vi "Setattribute_value.vi"(8 "error in (no error)":errorcluster, 10 "Set_Val":T1, 11 "OneOfTemplate in":refnum<class "niswitch_grpc_SetAttributeViInt32Request_attribute_value_enum.lvclass">) -> (0 "error out":errorcluster, 3 "OneOfTemplate out":refnum<class "niswitch_grpc_SetAttributeViInt32Request_attribute_value_enum.lvclass">)   [LabVIEW 2021, in "NI Switch_client.lvlib" / "niswitch_grpc_SetAttributeViInt32Request_attribute_value_enum.lvclass"]
uses:
  niswitch_grpc_SetAttributeViInt32Request_attribute_value_enum.lvclass
  niswitch_grpc_NiSwitchInt32AttributeValues.ctl
  niswitch_grpc_SetAttributeViInt32Request_attribute_value_enum.lvclass/niswitch_grpc_SetAttributeViInt32Request_attribute_value_enum.ctl
  NI Switch_client.lvlib
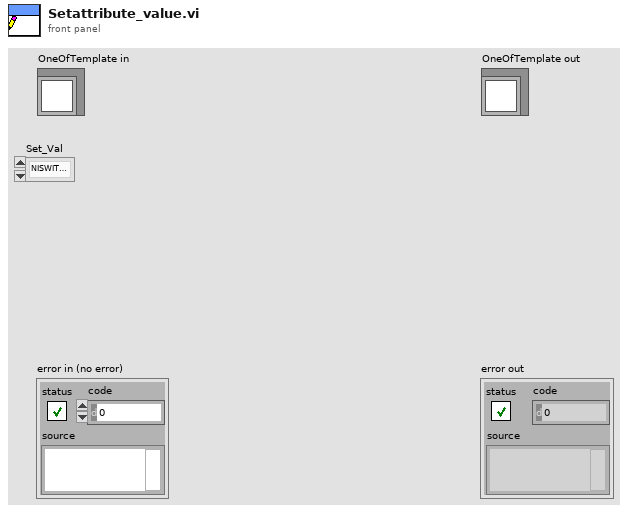
[diagram p1: front panel]
types:
  T1 = typedef "NI Switch_client.lvlib/niswitch_grpc_NiSwitchInt32AttributeValues.ctl" = enum32{"NISWITCH_INT32_UNSPECIFIED", "NISWITCH_INT32_HANDSHAKING_INITIATION_VAL_MEASUREMENT_DEVICE_INITIATED", "NISWITCH_INT32_HANDSHAKING_INITIATION_VAL_SWITCH_INITIATED", "NISWITCH_INT32_SCAN_ADVANCED_OUTPUT_VAL_NONE", "NISWITCH_INT32_SCAN_ADVANCED_OUTPUT_VAL_EXTERNAL", "NISWITCH_INT32_SCAN_ADVANCED_OUTPUT_VAL_TTL0", "NISWITCH_INT32_SCAN_ADVANCED_OUTPUT_VAL_TTL1", "NISWITCH_INT32_SCAN_ADVANCED_OUTPUT_VAL_TTL2", "NISWITCH_INT32_SCAN_ADVANCED_OUTPUT_VAL_TTL3", "NISWITCH_INT32_SCAN_ADVANCED_OUTPUT_VAL_TTL4", "NISWITCH_INT32_SCAN_ADVANCED_OUTPUT_VAL_TTL5", "NISWITCH_INT32_SCAN_ADVANCED_OUTPUT_VAL_TTL6", "NISWITCH_INT32_SCAN_ADVANCED_OUTPUT_VAL_TTL7", "NISWITCH_INT32_SCAN_ADVANCED_OUTPUT_VAL_PXI_STAR", "NISWITCH_INT32_SCAN_ADVANCED_OUTPUT_VAL_REARCONNECTOR", "NISWITCH_INT32_SCAN_ADVANCED_OUTPUT_VAL_FRONTCONNECTOR", "NISWITCH_INT32_SCAN_ADVANCED_OUTPUT_VAL_REARCONNECTOR_MODULE1", "NISWITCH_INT32_SCAN_ADVANCED_OUTPUT_VAL_REARCONNECTOR_MODULE2", "NISWITCH_INT32_SCAN_ADVANCED_OUTPUT_VAL_REARCONNECTOR_MODULE3", "NISWITCH_INT32_SCAN_ADVANCED_OUTPUT_VAL_REARCONNECTOR_MODULE4", "NISWITCH_INT32_SCAN_ADVANCED_OUTPUT_VAL_REARCONNECTOR_MODULE5", "NISWITCH_INT32_SCAN_ADVANCED_OUTPUT_VAL_REARCONNECTOR_MODULE6", "NISWITCH_INT32_SCAN_ADVANCED_OUTPUT_VAL_REARCONNECTOR_MODULE7", "NISWITCH_INT32_SCAN_ADVANCED_OUTPUT_VAL_REARCONNECTOR_MODULE8", "NISWITCH_INT32_SCAN_ADVANCED_OUTPUT_VAL_REARCONNECTOR_MODULE9", "NISWITCH_INT32_SCAN_ADVANCED_OUTPUT_VAL_REARCONNECTOR_MODULE10", "NISWITCH_INT32_SCAN_ADVANCED_OUTPUT_VAL_REARCONNECTOR_MODULE11", "NISWITCH_INT32_SCAN_ADVANCED_OUTPUT_VAL_REARCONNECTOR_MODULE12", "NISWITCH_INT32_SCAN_ADVANCED_OUTPUT_VAL_FRONTCONNECTOR_MODULE1", "NISWITCH_INT32_SCAN_ADVANCED_OUTPUT_VAL_FRONTCONNECTOR_MODULE2", "NISWITCH_INT32_SCAN_ADVANCED_OUTPUT_VAL_FRONTCONNECTOR_MODULE3", "NISWITCH_INT32_SCAN_ADVANCED_OUTPUT_VAL_FRONTCONNECTOR_MODULE4", "NISWITCH_INT32_SCAN_ADVANCED_OUTPUT_VAL_FRONTCONNECTOR_MODULE5", "NISWITCH_INT32_SCAN_ADVANCED_OUTPUT_VAL_FRONTCONNECTOR_MODULE6", "NISWITCH_INT32_SCAN_ADVANCED_OUTPUT_VAL_FRONTCONNECTOR_MODULE7", "NISWITCH_INT32_SCAN_ADVANCED_OUTPUT_VAL_FRONTCONNECTOR_MODULE8", "NISWITCH_INT32_SCAN_ADVANCED_OUTPUT_VAL_FRONTCONNECTOR_MODULE9", "NISWITCH_INT32_SCAN_ADVANCED_OUTPUT_VAL_FRONTCONNECTOR_MODULE10", "NISWITCH_INT32_SCAN_ADVANCED_OUTPUT_VAL_FRONTCONNECTOR_MODULE11", "NISWITCH_INT32_SCAN_ADVANCED_OUTPUT_VAL_FRONTCONNECTOR_MODULE12", "NISWITCH_INT32_SCAN_ADVANCED_POLARITY_VAL_RISING_EDGE", "NISWITCH_INT32_SCAN_ADVANCED_POLARITY_VAL_FALLING_EDGE", "NISWITCH_INT32_SCAN_MODE_VAL_NONE", "NISWITCH_INT32_SCAN_MODE_VAL_BREAK_BEFORE_MAKE", "NISWITCH_INT32_SCAN_MODE_VAL_BREAK_AFTER_MAKE", "NISWITCH_INT32_TRIGGER_INPUT_VAL_IMMEDIATE", "NISWITCH_INT32_TRIGGER_INPUT_VAL_EXTERNAL", "NISWITCH_INT32_TRIGGER_INPUT_VAL_SOFTWARE_TRIG", "NISWITCH_INT32_TRIGGER_INPUT_VAL_TTL0", "NISWITCH_INT32_TRIGGER_INPUT_VAL_TTL1", "NISWITCH_INT32_TRIGGER_INPUT_VAL_TTL2", "NISWITCH_INT32_TRIGGER_INPUT_VAL_TTL3", "NISWITCH_INT32_TRIGGER_INPUT_VAL_TTL4", "NISWITCH_INT32_TRIGGER_INPUT_VAL_TTL5", "NISWITCH_INT32_TRIGGER_INPUT_VAL_TTL6", "NISWITCH_INT32_TRIGGER_INPUT_VAL_TTL7", "NISWITCH_INT32_TRIGGER_INPUT_VAL_PXI_STAR", "NISWITCH_INT32_TRIGGER_INPUT_VAL_REARCONNECTOR", "NISWITCH_INT32_TRIGGER_INPUT_VAL_FRONTCONNECTOR", "NISWITCH_INT32_TRIGGER_INPUT_VAL_REARCONNECTOR_MODULE1", "NISWITCH_INT32_TRIGGER_INPUT_VAL_REARCONNECTOR_MODULE2", "NISWITCH_INT32_TRIGGER_INPUT_VAL_REARCONNECTOR_MODULE3", "NISWITCH_INT32_TRIGGER_INPUT_VAL_REARCONNECTOR_MODULE4", "NISWITCH_INT32_TRIGGER_INPUT_VAL_REARCONNECTOR_MODULE5", "NISWITCH_INT32_TRIGGER_INPUT_VAL_REARCONNECTOR_MODULE6", "NISWITCH_INT32_TRIGGER_INPUT_VAL_REARCONNECTOR_MODULE7", "NISWITCH_INT32_TRIGGER_INPUT_VAL_REARCONNECTOR_MODULE8", "NISWITCH_INT32_TRIGGER_INPUT_VAL_REARCONNECTOR_MODULE9", "NISWITCH_INT32_TRIGGER_INPUT_VAL_REARCONNECTOR_MODULE10", "NISWITCH_INT32_TRIGGER_INPUT_VAL_REARCONNECTOR_MODULE11", "NISWITCH_INT32_TRIGGER_INPUT_VAL_REARCONNECTOR_MODULE12", "NISWITCH_INT32_TRIGGER_INPUT_VAL_FRONTCONNECTOR_MODULE1", "NISWITCH_INT32_TRIGGER_INPUT_VAL_FRONTCONNECTOR_MODULE2", "NISWITCH_INT32_TRIGGER_INPUT_VAL_FRONTCONNECTOR_MODULE3", "NISWITCH_INT32_TRIGGER_INPUT_VAL_FRONTCONNECTOR_MODULE4", "NISWITCH_INT32_TRIGGER_INPUT_VAL_FRONTCONNECTOR_MODULE5", "NISWITCH_INT32_TRIGGER_INPUT_VAL_FRONTCONNECTOR_MODULE6", "NISWITCH_INT32_TRIGGER_INPUT_VAL_FRONTCONNECTOR_MODULE7", "NISWITCH_INT32_TRIGGER_INPUT_VAL_FRONTCONNECTOR_MODULE8", "NISWITCH_INT32_TRIGGER_INPUT_VAL_FRONTCONNECTOR_MODULE9", "NISWITCH_INT32_TRIGGER_INPUT_VAL_FRONTCONNECTOR_MODULE10", "NISWITCH_INT32_TRIGGER_INPUT_VAL_FRONTCONNECTOR_MODULE11", "NISWITCH_INT32_TRIGGER_INPUT_VAL_FRONTCONNECTOR_MODULE12", "NISWITCH_INT32_TRIGGER_INPUT_POLARITY_VAL_RISING_EDGE", "NISWITCH_INT32_TRIGGER_INPUT_POLARITY_VAL_FALLING_EDGE", "NISWITCH_INT32_WIRE_MODE_VAL_1_WIRE", "NISWITCH_INT32_WIRE_MODE_VAL_2_WIRE", "NISWITCH_INT32_WIRE_MODE_VAL_4_WIRE"}
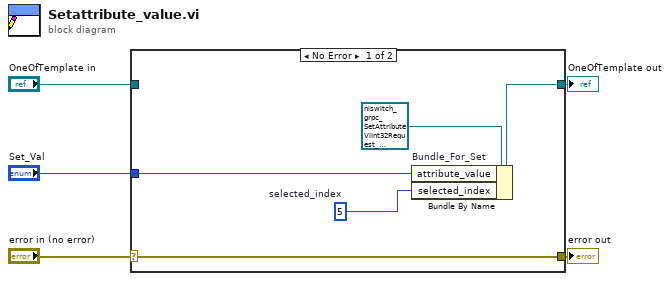
[diagram p0: block diagram]
diagram:
  n1 = case shown="No Error" "error in (no error)" {
    selector: "error in (no error)" -> [w10 w11]
    tunnel: [w10 w11] -> w4
    tunnel: [w9 w12] -> w2
    tunnel: "OneOfTemplate in" -> [_ w12]
    tunnel: "Set_Val" -> [w8 _]
    frame No Error {
      w7 = 5  # selected_index
      n2 = Bundle By Name "Bundle_For_Set"(cluster=refnum<class "niswitch_grpc_SetAttributeViInt32Request_attribute_value_enum.lvclass"> refnum ("OneOfTemplate in"), "attribute_value"=w8, "selected_index"=w7) -> (w9:refnum<class "niswitch_grpc_SetAttributeViInt32Request_attribute_value_enum.lvclass">)
    }
    frame Error {
    }
  }
  "error out" <- w4
  "OneOfTemplate out" <- w2
